vi "DSF.Engine.Plugin.Command.Unbundle.vi"(8 "error in (no error)":errorcluster, 10 "command":T3, 11 "Plugin in":refnum<class "DSF.Engine.Plugin.lvclass">) -> (0 "error out":errorcluster, 1 "command":T1, 2 "command parameters":T2, 3 "Plugin out":refnum<class "DSF.Engine.Plugin.lvclass">)   [LabVIEW 2017, in "DSF.Engine.lvlib" / "DSF.Engine.Plugin.lvclass"]
uses:
  DSF.Engine.Plugin.lvclass
  Interface/DSF.Engine.Interface.Plugin.Command Data.ctl
  Interface/DSF.Engine.Interface.Plugin.Command.ctl
  Interface/DSF.Engine.Interface.Plugin.Command Parameters.ctl
  Interface/DSF.Engine.Interface.Plugin.lvclass
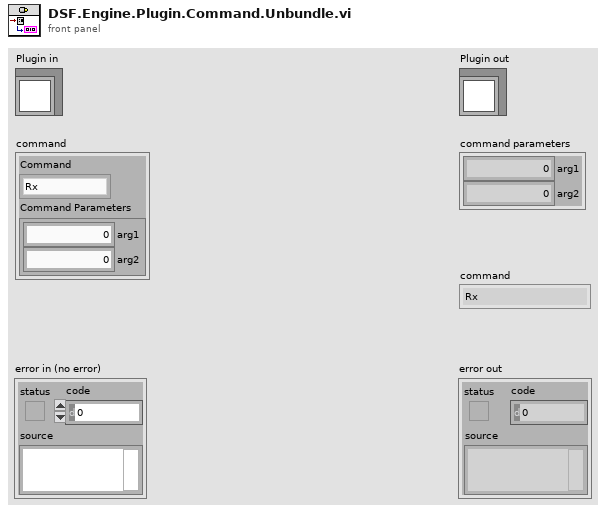
[diagram p1: front panel]
types:
  T1 = typedef "DSF.Engine.lvlib/DSF.Engine.Interface.Plugin.lvclass/DSF.Engine.Interface.Plugin.Command.ctl" = enum8{"Rx", "Tx", "Shutdown"}
  T2 = typedef "DSF.Engine.lvlib/DSF.Engine.Interface.Plugin.lvclass/DSF.Engine.Interface.Plugin.Command Parameters.ctl" = cluster{"arg1":u64, "arg2":u64}
  T3 = typedef "DSF.Engine.lvlib/DSF.Engine.Interface.Plugin.lvclass/DSF.Engine.Interface.Plugin.Command Data.ctl" = cluster{"Command":T1, "Command Parameters":T2}
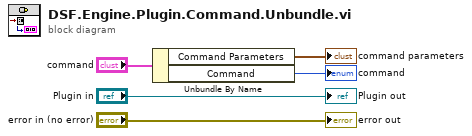
[diagram p0: block diagram]
diagram:
  n1 = Unbundle By Name("command") -> ("Command Parameters"=→"command parameters":T2, "Command"=→"command":T1)
  "error out" <- "error in (no error)"
  "Plugin out" <- "Plugin in"
